vi "Configure Data Marker [DM].vi"(6 "Destination Terminal (None)":string(combo) caption="destination terminal (None)", 7 "Bit Position":i32 caption="bit position" format="%.0g", 8 "error in (no error)":errorcluster, 9 "Marker Name (\"\")":string caption="marker name (\"\")", 10 "Source Channel (\"\")":string="CHANNEL1" caption="source channel (\"CHANNEL1\")", 11 "CS++Fgen in":refnum<class "CS++Fgen.lvclass">) -> (0 "error out":errorcluster, 3 "CS++Fgen out":refnum<class "CS++Fgen.lvclass">)   [LabVIEW 2013, in "CS++Fgen.lvlib" / "CS++Fgen.lvclass"]
doc: "This VI configures the common data marker properties. These properties are the data marker source channel, bit position, and destination.\n \nNote:\n\n(1) This VI is part of the IviFgenDataMarker [DM] extension group."
uses:
  CS++Fgen.lvclass
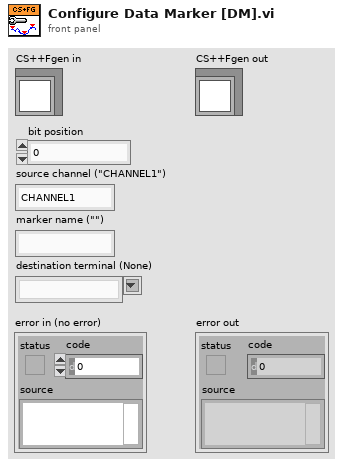
[diagram p1: front panel]
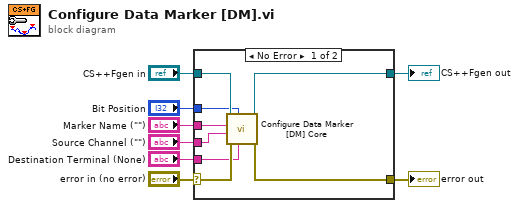
[diagram p0: block diagram]
diagram:
  n1 = case shown="No Error" "error in (no error)" {
    selector: "error in (no error)" -> [w14 w18]
    tunnel: [w13 w18] -> w7
    tunnel: [w15 w17] -> w5
    tunnel: "CS++Fgen in" -> [w16 w17]
    tunnel: "Bit Position" -> [w10 _]
    tunnel: "Marker Name (\"\")" -> [w12 _]
    tunnel: "Source Channel (\"\")" -> [w11 _]
    tunnel: "Destination Terminal (None)" -> [w9 _]
    frame No Error {
      n2 = call-dynamic "Configure Data Marker [DM] Core.vi"("Destination Terminal (None)"=w9, "Bit Position"=w10, "error in (no error)"=w14, "Marker Name (\"\")"=w11, "Source Channel (\"\")"=w12, "CS++Fgen in"=w16) -> ("error out"=w13:errorcluster, "CS++Fgen out"=w15:refnum<class "CS++Fgen.lvclass">)  [unwired: 4 in]
    }
    frame Error {
    }
  }
  "error out" <- w7
  "CS++Fgen out" <- w5
